vi "Alarma_AVANZADO.vi"() -> ()   [LabVIEW 2020]
panel:
  out "Waveform Chart":dbl(graph)
  out "Text 3":string
  out "Text 2":string
  out "Text 1":string
  in  "Limite Max":dbl(slide) scale=0.0..100.0
  in  "Limite Min":dbl(slide) scale=0.0..100.0
  out "Alarma 3":bool
  out "Alarma 2":bool
  out "Alarma 1":bool
  in  "Temp3":u16(slide) scale=0.0..100.0
  in  "Temp2":i16(slide) scale=0.0..100.0
  in  "Temp1":dbl(slide) scale=0.0..100.0
  # "Indicador de Alarmas"
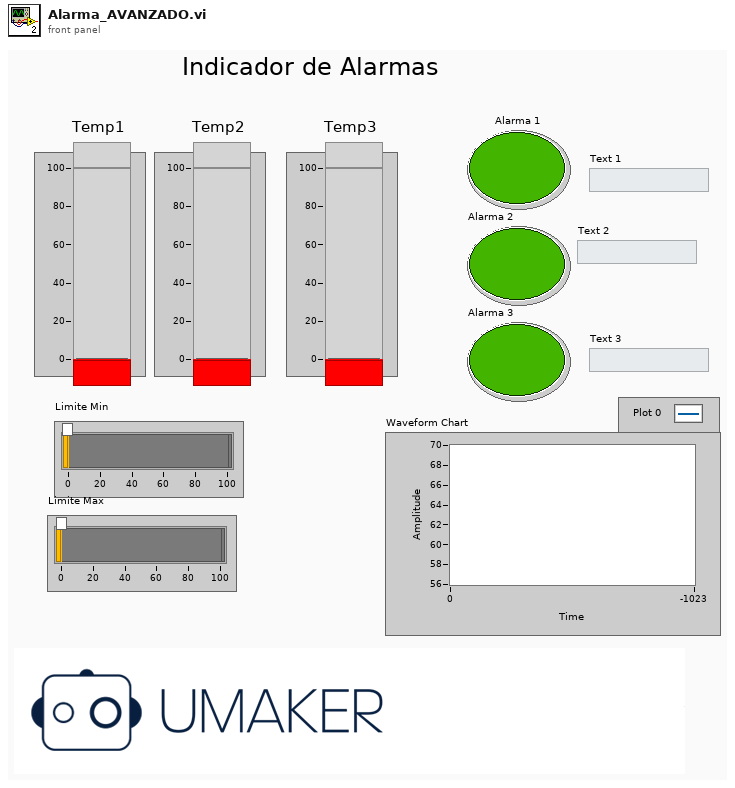
[diagram p1: front panel]
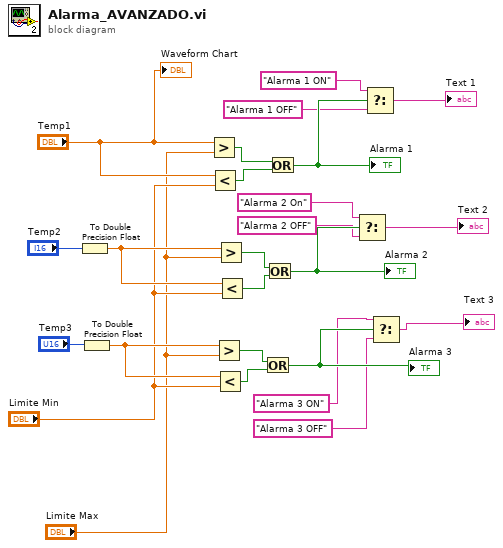
[diagram p0: block diagram]
diagram:
  n1 = To Double Precision Float(number="Temp2") -> (double precision float=w23:dbl)
  n2 = To Double Precision Float(number="Temp3") -> (double precision float=w22:dbl)
  n3 = Greater?(x="Temp1", y="Limite Max") -> (0:w21:bool)
  n4 = Less?(x="Temp1", y="Limite Min") -> (x < y?=w20:bool)
  n5 = Greater?(x=w22, y="Limite Max") -> (0:w16:bool)
  n6 = Less?(x=w22, y="Limite Min") -> (x < y?=w19:bool)
  n7 = Greater?(x=w23, y="Limite Max") -> (0:w18:bool)
  n8 = Less?(x=w23, y="Limite Min") -> (x < y?=w17:bool)
  n9 = Or(x=w16, y=w19) -> (x .or. y?=w13:bool)
  "Alarma 3" <- w13
  n10 = Or(x=w18, y=w17) -> (x .or. y?=w14:bool)
  "Alarma 2" <- w14
  n11 = Or(x=w21, y=w20) -> (x .or. y?=w15:bool)
  "Alarma 1" <- w15
  n12 = Select(t="Alarma 2 On", s=w14, f="Alarma 2 OFF") -> (s? t:f=→"Text 2":string)
  n13 = Select(t="Alarma 1 ON", s=w15, f="Alarma 1 OFF") -> (s? t:f=→"Text 1":string)
  n14 = Select(t="Alarma 3 ON", s=w13, f="Alarma 3 OFF") -> (s? t:f=→"Text 3":string)
  "Waveform Chart" <- "Temp1"
